vi "DistBetweenPoints.vi"(1 "UTM Location 2":T1 {"North" format="%#_10f"; "East" format="%#_8f"}, 2 "UTM Location":T1 {"North" format="%#_10f"; "East" format="%#_8f"}) -> (0 "Numeric":dbl)   [LabVIEW 2012]
doc: "Calcs Distance between two UTM Locations. Does not take into account timezone or hemisphere."
uses:
  Data/TypeDefs/UTM Location.ctl
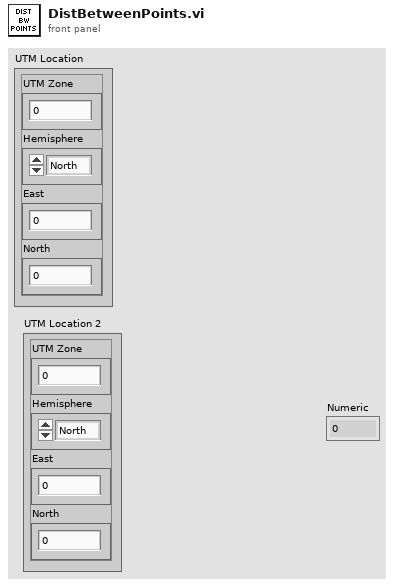
[diagram p1: front panel]
types:
  T1 = typedef "UTM Location.ctl" = cluster{"UTM Zone":dbl, "Hemisphere":enum16{"North", "South"}, "East":dbl, "North":dbl}
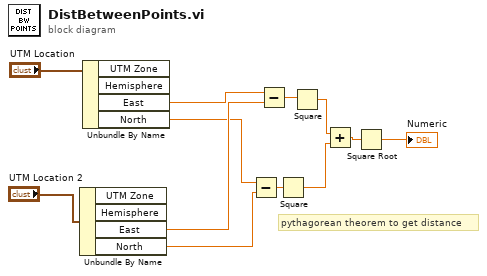
[diagram p0: block diagram]
diagram:
  # "pythagorean theorem to get distance"
  n1 = Unbundle By Name("UTM Location 2") -> ("East"=w9:dbl, "North"=w7:dbl)  [unwired: 2 out]
  n2 = Unbundle By Name("UTM Location") -> ("East"=w10:dbl, "North"=w8:dbl)  [unwired: 2 out]
  n3 = Subtract(x=w8, y=w7) -> (x-y=w5:dbl)
  n4 = Subtract(x=w10, y=w9) -> (x-y=w6:dbl)
  n5 = Square(x=w5) -> (x^2=w3:dbl)
  n6 = Square(x=w6) -> (x^2=w4:dbl)
  n7 = Add(x=w4, y=w3) -> (x+y=w2:dbl)
  n8 = Square Root(x=w2) -> (sqrt(x)=→"Numeric":dbl)
